vi "_save_csv_Freq.vi"(7 "delimiter (\\t)":string="SingleCh_", 11 "Data":dbl[][](array[numeric])) -> (3 "FileName":string)   [LabVIEW 2023]
uses:
  <vilib>/Utility/file.llb/Write Delimited Spreadsheet (string).vi
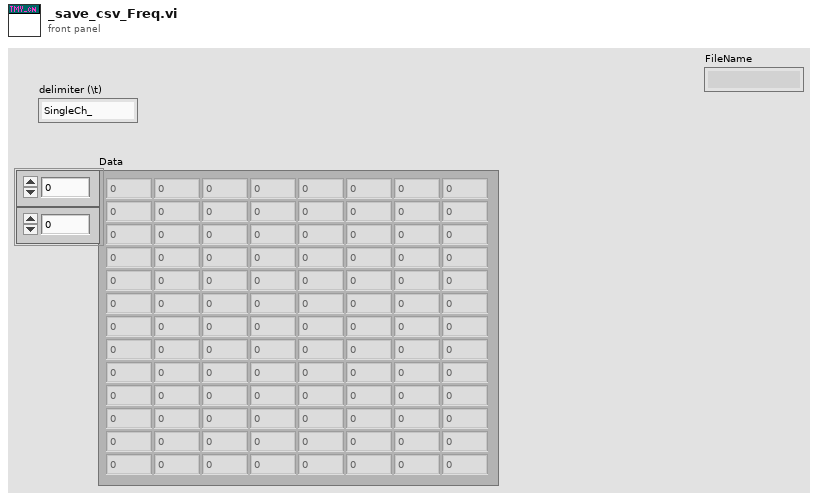
[diagram p1: front panel]
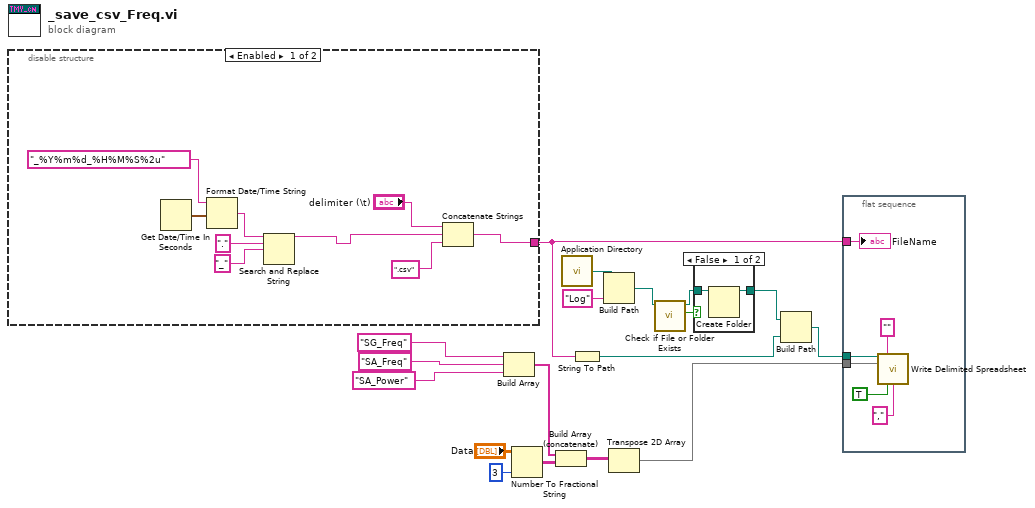
[diagram p0: block diagram]
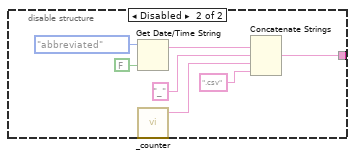
[diagram p3: hidden frame]
diagram:
  n1 = disable-structure shown="Enabled" {
    disable-tunnel: [w26 w28] -> w15
    frame Enabled {
      n2 = Get Date/Time In Seconds() -> (seconds since 1Jan1904=w24:timestamp)
      n3 = Format Date/Time String(time format string (%c)="_%Y%m%d_%H%M%S%2u", seconds (now)=w24) -> (date/time string=w22:string)  [unwired: 1 in]
      n4 = Search and Replace String(input string=w22, search string=".", replace string="_") -> (result string=w19:string)  [unwired: 5 in, 3 out]
      n5 = Concatenate Strings("delimiter (\\t)", w19, ".csv" ("delimiter (\\t)")) -> (w26:string)
    }
    frame Disabled {
      n6 = Get Date/Time String(date format (0)=enum16{"short", "long", "abbreviated"}."abbreviated", want seconds? (F)=FALSE) -> (date string=w35:string)  [unwired: 1 in, 1 out]
      n7 = call "_counter.vi"() -> ("out_count"=w29:string)  [unwired: 5 in]
      n8 = Concatenate Strings(w35, "_" ("delimiter (\\t)"), w29, ".csv" ("delimiter (\\t)")) -> (w28:string, w30:string)
    }
  }
  n9 = Build Array("SG_Freq", "SA_Freq", "SA_Power") -> (w4:string[])
  n10 = Number To Fractional String(number="Data", precision (6)=i16 3) -> (F-format string=w5:string[][])  [unwired: 2 in]
  n11 = Build Array (concatenate)(w4, w5) -> (w3:string[][])
  n12 = call <vilib>:"Application Directory.vi"() -> ("Application Directory"=w14:path)
  n13 = String To Path(string=w15) -> (path=w17:path)
  n14 = Build Path(base path=w14, name or relative path="Log") -> (appended path=w11:path)
  n15 = Transpose 2D Array(2D array=w3) -> (transposed array=w2:string[][])
  n16 = call <vilib>:"Check if File or Folder Exists.vi"("path"=w11) -> ("file or folder exists?"=w13:bool, "dup path"=w12:path)  [unwired: 8 in, 1 out]
  n17 = case shown="False" w13 {
    tunnel: w12 -> [w37 w38]
    tunnel: [w36 w38] -> w10
    frame False {
      n18 = Create Folder(path (use dialog)=w37) -> (created path=w36:path)  [unwired: 2 in, 2 out]
    }
    frame True {
    }
  }
  n19 = Build Path(base path=w10, name or relative path=w17) -> (appended path=w16:path)
  n20 = flat-sequence {
    tunnel: w16 -> [w43]
    tunnel: w15 -> [w41]
    tunnel: w2 -> [w39]
    frame #0 {
      n21 = call-poly <vilib>:"Write Delimited Spreadsheet.vi"("file path (dialog if empty)"=w43, "format (%s)"="" ("format (%.3f)"), "2D data"=w39, "transpose? (no:F)"=TRUE, "delimiter (\\t)"="," ("delimiter (\\t)")) -> ()  [unwired: 9 in, 2 out]
      "FileName" <- w41
    }
  }
